vi "报警信息字段定义.vi"(7 "table输入":string, 11 "data in":T1) -> (1 "table输出":string, 2 "columns":string[](array[string]), 3 "data out":T1)   [LabVIEW 2016, in "斯坦道CODMn.lvlib"]
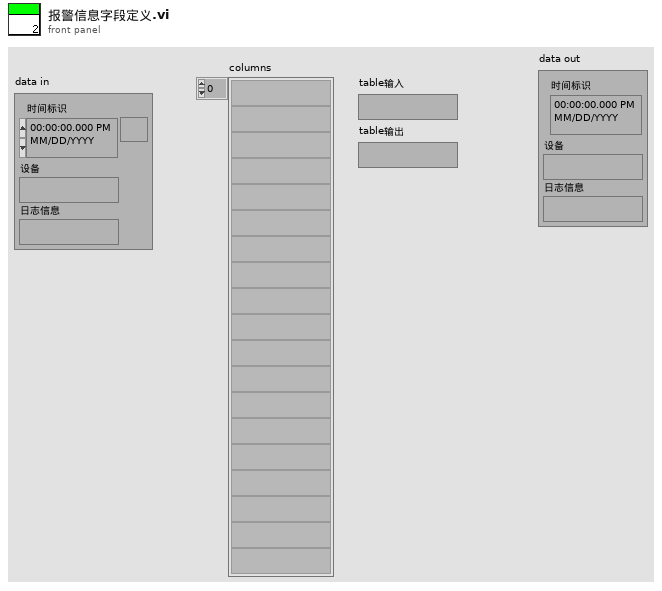
[diagram p1: front panel]
types:
  T1 = cluster{"时间标识":timestamp, "设备":string, "日志信息":string}
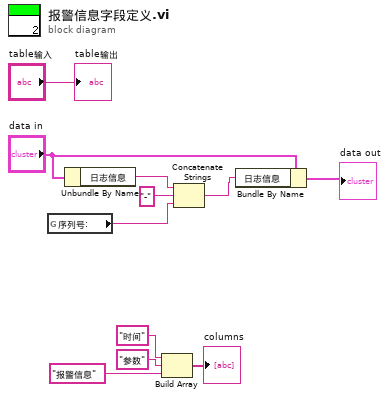
[diagram p0: block diagram]
diagram:
  n1 = global read "COD内部交互全局.vi" "序列号:"() -> (w1:string)
  n2 = Unbundle By Name("data in") -> ("日志信息"=w4:string)
  n3 = Build Array("时间", "参数" ("元素"), "报警信息") -> (→"columns":string[])
  n4 = Concatenate Strings(w4, "-" ("字符串"), w1) -> (w3:string)
  n5 = Bundle By Name(cluster="data in", "日志信息"=w3) -> (→"data out":T1)
  "table输出" <- "table输入"
